vi "Read-Save DefaultSerialPort.vi"(6 "Task":enum16{"Save", "Read"}(ring)=enum."Read", 10 "steps per degree":dbl=1.67, 11 "VISA":refnum<visa-resource-name>) -> (0 "Pref Path":path, 2 "steps per degree out":dbl=1.67, 3 "VISA out":refnum<visa-resource-name>)   [LabVIEW 2022 SP3]
panel:
  out "text":string
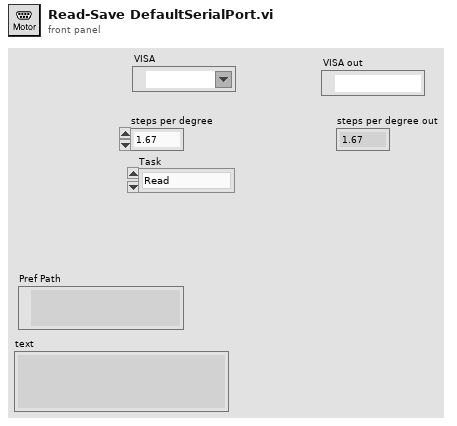
[diagram p1: front panel]
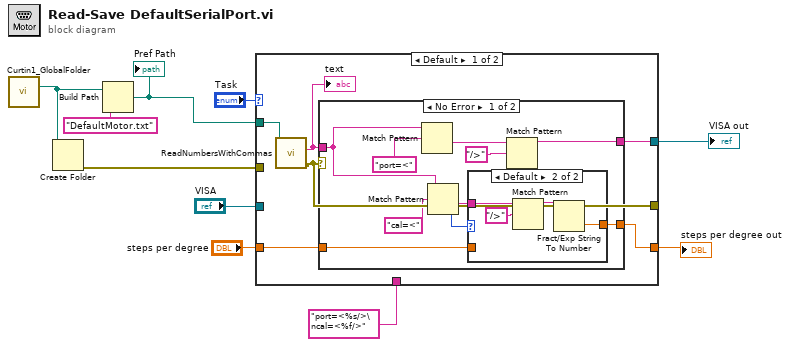
[diagram p0: block diagram]
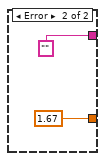
[diagram p3: hidden frame]
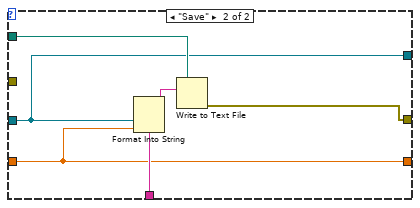
[diagram p4: hidden frame]
diagram:
  n1 = call "Curtin1_GlobalFolder.vi"() -> ("LabVIEW Data Path"=w5:path)  [unwired: 1 in, 1 out]
  n2 = Create Folder(path (use dialog)=w5) -> (error out=w6:errorcluster)  [unwired: 2 in, 2 out]
  n3 = Build Path(base path=w5, name or relative path="DefaultMotor.txt") -> (appended path=w9:path)
  "Pref Path" <- w9
  n4 = case shown="Default" "Task" {
    tunnel: "VISA" -> [_ w36]
    tunnel: w9 -> [w15 w39]
    tunnel: [w13 w37] -> _
    tunnel: [w16 w36] -> w3
    tunnel: w6 -> [_ _]
    tunnel: "port=<%s/>\ncal=<%f/>" ("format string") -> [_ w35]
    tunnel: "steps per degree" -> [w11 w34]
    tunnel: [w12 w34] -> w1
    frame Default {
      n5 = call "ReadNumbersWithCommas.vi"("file (use dialog)"=w15) -> ("error out"=w13:errorcluster, "text"=w14:string)  [unwired: 7 in, 2 out]
      "text" <- w14
      n6 = case shown="No Error" w13 {
        tunnel: [w24 "" ("Notes")] -> w16
        tunnel: w14 -> [w20 _]
        tunnel: [w19 1.67] -> w12
        tunnel: w11 -> [w17 _]
        frame No Error {
          n7 = Match Pattern(string=w20, regular expression="port=<" ("format string")) -> (after substring=w26:string)  [unwired: 1 in, 3 out]
          n8 = Match Pattern(string=w20, regular expression="cal=<" ("format string")) -> (after substring=w22:string, offset past match=w18:i32)  [unwired: 1 in, 2 out]
          n9 = case shown="Default" w18 {
            tunnel: w22 -> [_ w30]
            tunnel: [w27 w28] -> w19
            tunnel: w17 -> [w27 _]
            frame -1 {
            }
            frame Default {
              n10 = Match Pattern(string=w30, regular expression="/>" ("format string")) -> (before substring=w29:string)  [unwired: 1 in, 3 out]
              n11 = Fract/Exp String To Number(string=w29) -> (number=w28:dbl)  [unwired: 3 in, 1 out]
            }
          }
          n12 = Match Pattern(string=w26, regular expression="/>" ("format string")) -> (before substring=w24:string)  [unwired: 1 in, 3 out]
        }
        frame Error {
        }
      }
    }
    frame "Save" {
      n13 = Format Into String(format string=w35, w36, w34) -> (resulting string=w38:string)  [unwired: 2 in, 1 out]
      n14 = Write to Text File(file (use dialog)=w39, text=w38) -> (error out=w37:errorcluster)  [unwired: 2 in, 2 out]
    }
  }
  "VISA out" <- w3
  "steps per degree out" <- w1
